vi "Script_New.vi"(1 "Script name":string, 5 "error in":errorcluster, 7 "Working Script":path, 9 "Saved Tree":T2[](array[typedef]), 10 "Config Cluster":T1) -> (11 "Saved Tree out":T2[](array[typedef]), 13 "Working Script out":path, 15 "Script name out":string, 19 "error out":errorcluster)   [LabVIEW 2010]
uses:
  ScriptStepTypeDef.ctl
  Config cluster.ctl
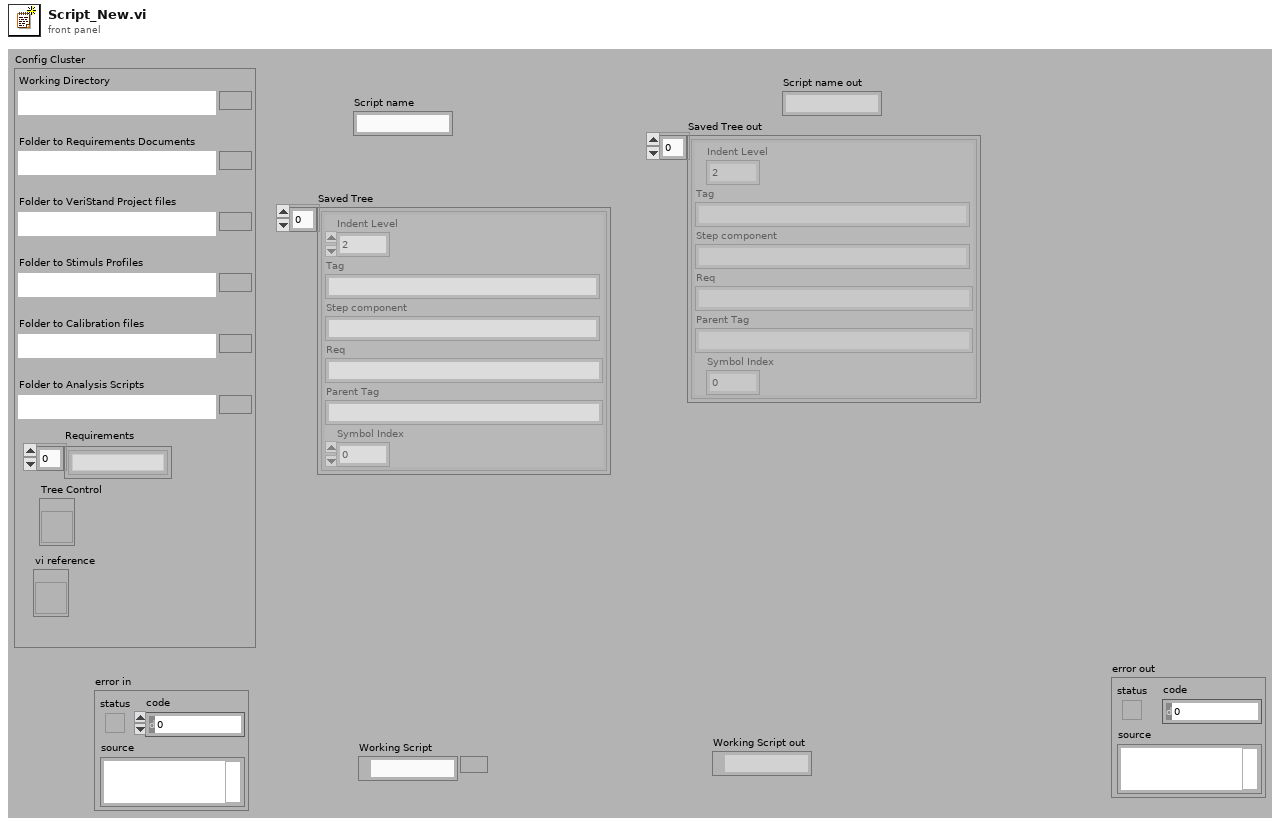
[diagram p1: front panel]
types:
  T1 = typedef "Config cluster.ctl" = cluster{"Working Directory":path, "Folder to Requirements Documents":path, "Folder to VeriStand Project files":path, "Folder to Stimuls Profiles":path, "Folder to Calibration files":path, "Folder to Analysis Scripts":path, "Requirements":string[], "Tree Control":refnum<vi>, "vi reference":refnum<vi>}
  T2 = typedef "ScriptStepTypeDef.ctl" = cluster{"Indent Level":i32, "Tag":string, "Step component":string, "Req":string, "Parent Tag":string, "Symbol Index":i32}
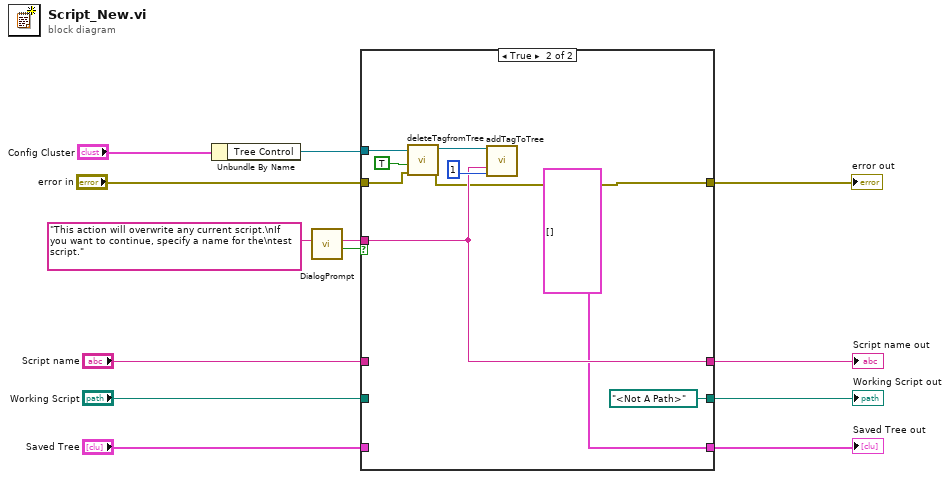
[diagram p0: block diagram]
diagram:
  n1 = Unbundle By Name("Config Cluster") -> ("Tree Control"=w6:refnum<vi>)
  n2 = call "DialogPrompt.vi"("Dialog prompt"="This action will overwrite any current script.\nIf you want to continue, specify a name for the\ntest script." ("message")) -> ("OK out"=w3:bool, "Usert Txt(out)"=w4:string)  [unwired: 9 in]
  n3 = case shown="True" w3 {
    tunnel: w4 -> [_ w21]
    tunnel: w6 -> [_ w23]
    tunnel: "error in" -> [w14 w22]
    tunnel: "Script name" -> [w17 _]
    tunnel: [w17 w21] -> w9
    tunnel: "Working Script" -> [w16 _]
    tunnel: [w16 path "<Not A Path>" ("selected path")] -> w11
    tunnel: "Saved Tree" -> [w15 _]
    tunnel: [w15 T2[] [] ("Steps with Params")] -> w13
    tunnel: [w14 w18] -> w1
    frame False {
    }
    frame True {
      n4 = call "deleteTagfromTree.vi"("error in (no error)"=w22, "Delete Children?"=TRUE, "Tree Ref"=w23) -> ("error out"=w18:errorcluster, "Tree ref out"=w25:refnum<vi>)  [unwired: 7 in]
      n5 = call "addTagToTree.vi"("Tree ref"=w25, "new tag"=w21, "Symbol"=1) -> ()  [unwired: 12 in, 1 out]
    }
  }
  "Saved Tree out" <- w13
  "Working Script out" <- w11
  "Script name out" <- w9
  "error out" <- w1
